vi "Pre Launch Init.vi"(11 "Common in":refnum<class "Common.lvclass">) -> (0 "error out":errorcluster, 3 "Common out":refnum<class "Common.lvclass">)   [LabVIEW 2021, in "Common.lvlib" / "Common.lvclass"]
doc: "(<B>Filename</B>: Actor Framework.lvlib:Actor.lvclass:Pre Launch Init.vi)\n\nDefines behavior that occurs after the Launch Nested Actor method is invoked but before the actor's Actor Core method begins running.\n\nBy default, this method does nothing. A descendant class may override it to define behavior."
uses:
  Common.lvclass
  Common.lvclass/Common.ctl
  <vilib>/ActorFramework/Actor/Actor.lvclass
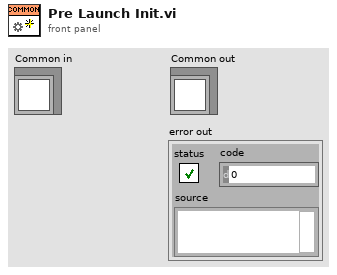
[diagram p1: front panel]
types:
  T1 = cluster{"message":string, "payload":string, "Time Stamp":timestamp}
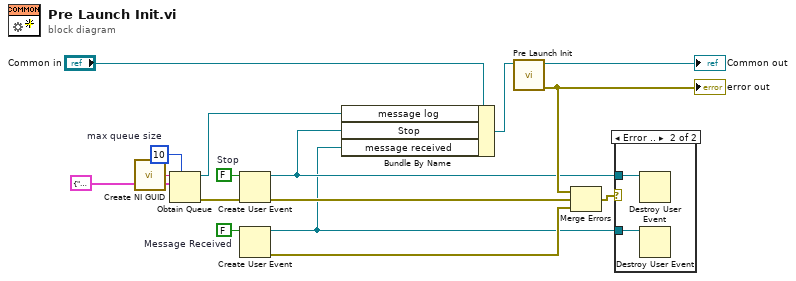
[diagram p0: block diagram]
diagram:
  w3 = FALSE  # Message Received
  w8 = 10  # max queue size
  w15 = FALSE  # Stop
  n1 = call <vilib>:"Create NI GUID.vi"() -> ("NI GUID"=w7:string)
  n2 = Obtain Queue(max queue size (-1, unlimited)=w8, name (unnamed)=w7, element data type=T1 {"message"="", "payload"="", "Time Stamp"=timestamp(0 s since 1904-01-01)}) -> (queue out=w4:refnum<queue>, error out=w6:errorcluster)  [unwired: 2 in, 1 out]
  n3 = Create User Event(user event datatype=w15, error in=w6) -> (user event=w9:refnum<user-event>, error out=w12:errorcluster)
  n4 = Create User Event(user event datatype=w3) -> (user event=w1:refnum<user-event>, error out=w2:errorcluster)  [unwired: 1 in]
  n5 = Bundle By Name(cluster="Common in", "message log"=w4, "Stop"=w9, "message received"=w1) -> (w13:refnum<class "Common.lvclass">)
  n6 = call-parent "Pre Launch Init.vi"("Actor in"=w13) -> ("error out"=w11:errorcluster, "Actor out"=→"Common out":refnum<class "Common.lvclass">)  [unwired: 9 in]
  "error out" <- w11
  n7 = Merge Errors(w11, w12, w2) -> (w10:errorcluster)
  n8 = case shown="Error .." w10 {
    tunnel: w9 -> [_ w18]
    tunnel: w1 -> [_ w17]
    frame No Error {
    }
    frame Error {
      n9 = Destroy User Event(user event=w18) -> ()  [unwired: 1 in, 1 out]
      n10 = Destroy User Event(user event=w17) -> ()  [unwired: 1 in, 1 out]
    }
  }
